vi "S2C_CMD_ShowCommand.vi"(7 "Error In":errorcluster, 10 "Row":i32, 11 "Data In":string[][](array[string])) -> (3 "Data Out":string[][](array[string]), 5 "Error Out":errorcluster)   [LabVIEW 2015]
doc: "Allows for the selection of available commands and parameters contained within a driver specific file."
panel:
  in  "Return":u16(ring) caption="Return Values"
  out "DriverText":string
  in  "Done":bool
  in  "Cmd":u16(ring) caption="Test"
  out "Init":bool
  in  "Params":i32(listbox) caption="Command"
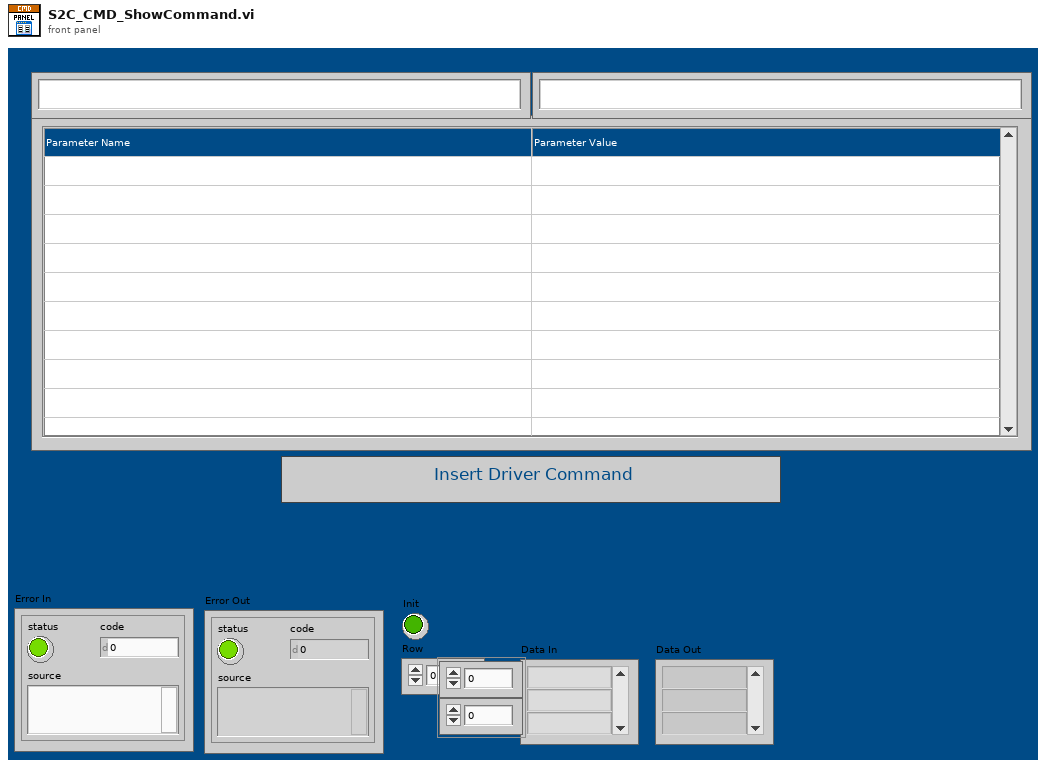
[diagram p1: front panel]
types:
  T1 = cluster{"Function":string, "Command":string, "Return":string, "Settings":string}
  T2 = typedef "LVPoint32TypeDef.ctl" = cluster{"Horizontal":i32, "Vertical":i32}
  T3 = typedef "LVRowAndColumnTypeDef.ctl" = cluster{"Row":i32, "Column":i32}
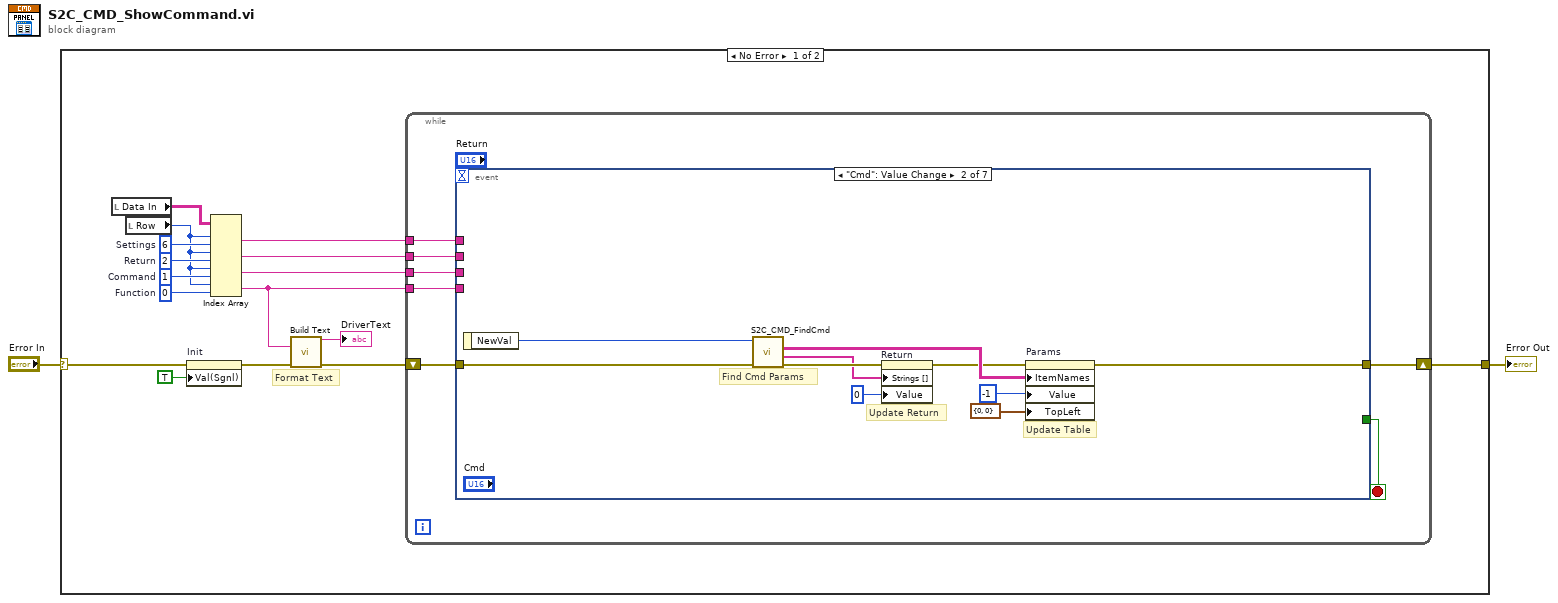
[diagram p0: block diagram]
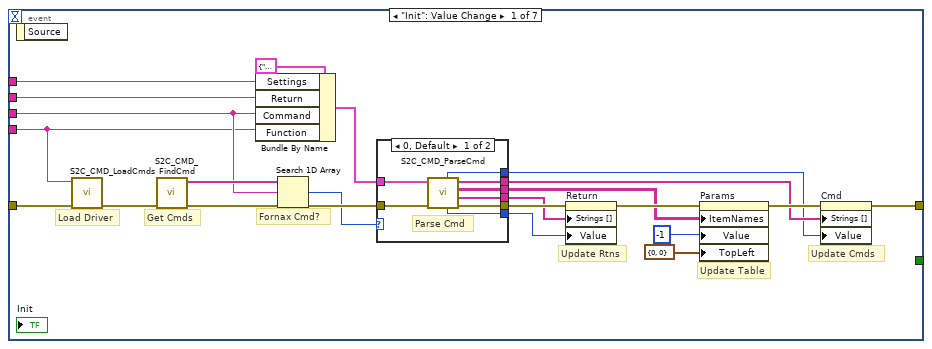
[diagram p2: hidden frame]
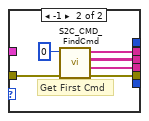
[diagram p3: hidden frame]
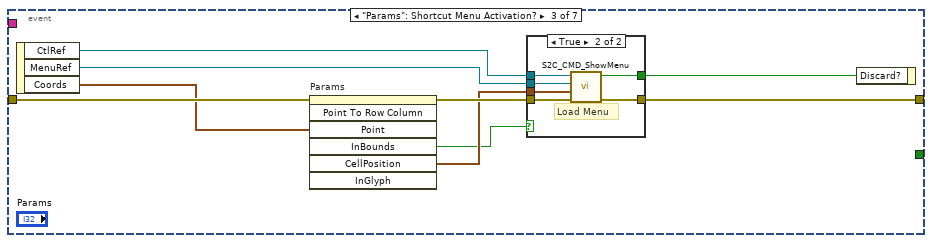
[diagram p4: hidden frame]
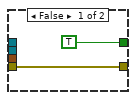
[diagram p5: hidden frame]
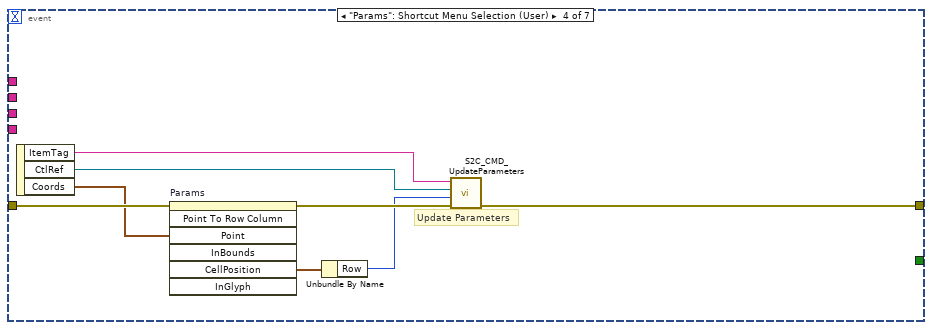
[diagram p6: hidden frame]
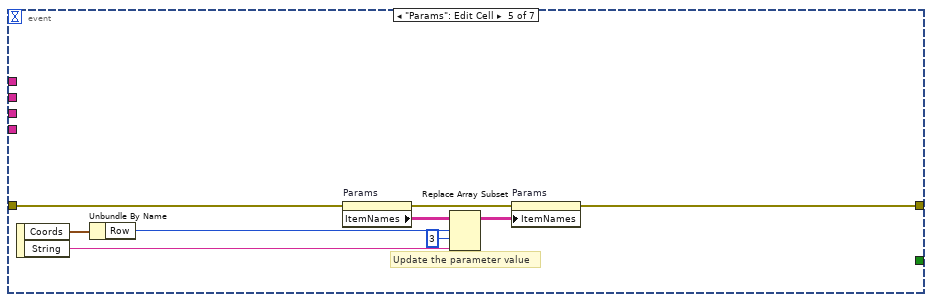
[diagram p7: hidden frame]
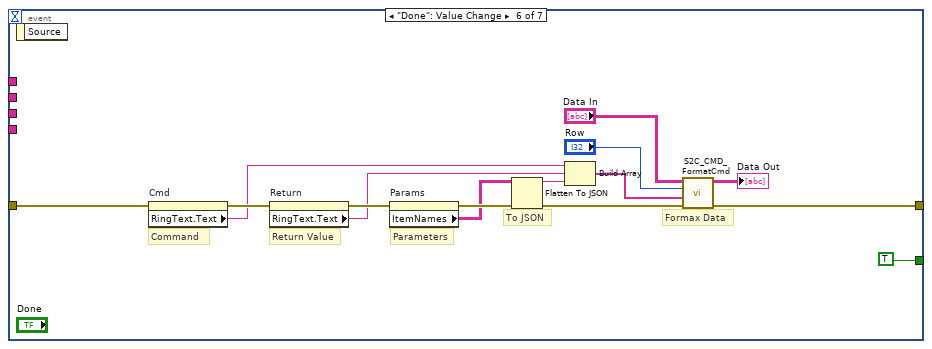
[diagram p8: hidden frame]
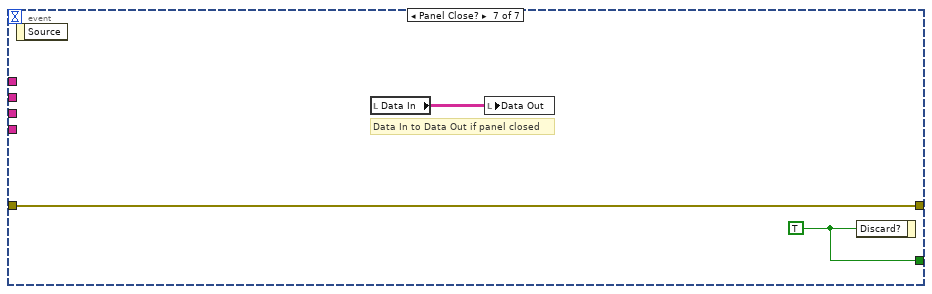
[diagram p9: hidden frame]
diagram:
  n1 = case shown="No Error" "Error In" {
    selector: "Error In" -> [w13 w124]
    tunnel: [w17 w124] -> w1
    frame No Error {
      w5 = 0  # Function
      w7 = 1  # Command
      w9 = 2  # Return
      w10 = 6  # Settings
      # "Format Text"
      n2 = local read "Data In"() -> (w15:string[][])
      n3 = local read "Row"() -> (w6:i32)
      n4 = property on="Init" class="Bool (strict)"(error in=w13, "Val(Sgnl)"=TRUE ("Value (Signaling)")) -> (error out=w12:errorcluster)  [unwired: 1 in, 1 out]
      n5 = Index Array(array=w15, index (row) #1=w6, index (col) #1=w10, index (row) #2=w6, index (col) #2=w9, index (row) #3=w6, index (col) #3=w7, index (row) #4=w6, index (col) #4=w5) -> (element #1=w14:string, element #2=w8:string, element #3=w3:string, element #4=w4:string)
      n6 = call "Build Text"("Driver"=w4, "error in (no error)"=w12) -> ("Result"=→"DriverText":string, "error out"=w11:errorcluster)  [unwired: 12 in]
      n7 = while {
        shift-right: [w24] -> w17
        shift-left: w11 -> [w25]
        tunnel: w14 -> [w22]
        tunnel: w8 -> [w21]
        tunnel: w4 -> [w20]
        tunnel: w3 -> [w19]
        stop <- w23 stop-if-true
        n8 = event shown="[1] \"Cmd\": Value Change" {
          selector: _ -> [_ _ _ _ _ _ _]
          dyn-events: _ -> [_ _ _ _ _ _ _]
          timeout: _ -> [_ _ _ _ _ _ _]
          tunnel: w25 -> [w41 w69 w80 w95 w104 w119 w123]
          tunnel: [w35 w70 w74 w93 w105 w108 w123] -> w24
          tunnel: [_ _ _ _ _ TRUE w122] -> w23
          tunnel: w22 -> [w31 _ _ _ _ _ _]
          tunnel: w21 -> [w30 _ _ _ _ _ _]
          tunnel: w20 -> [w28 _ _ _ _ _ _]
          tunnel: w19 -> [w29 _ _ _ _ _ _]
          event "Init": Value Change {
            # "Update Cmds"
            # "Load Driver"
            # "Fornax Cmd?"
            # "Get Cmds"
            # "Update Table"
            # "Update Rtns"
            n9 = event-data() -> ()  [unwired: 1 in, 1 out]
            n10 = call "S2C_CMD_LoadCmds.vi"("Error In"=w41, "Driver"=w28) -> ("Error Out"=w40:errorcluster)  [unwired: 9 in]
            n11 = call "S2C_CMD_FindCmd.vi"("Error In"=w40) -> ("Error Out"=w43:errorcluster, "AllCmds"=w34:string[])  [unwired: 7 in, 2 out]
            n12 = Bundle By Name(cluster=T1 {"Function"="", "Command"="", "Return"="", "Settings"=""}, "Settings"=w31, "Return"=w30, "Command"=w29, "Function"=w28) -> (w27:T1)
            n13 = Search 1D Array(1D array=w34, element=w29) -> (index of element=w42:i32)  [unwired: 1 in]
            n14 = case shown="0, Default" w42 {
              tunnel: w43 -> [w55 w61]
              tunnel: [w48 w56] -> w36
              tunnel: [w54 w59] -> w44
              tunnel: [w49 w57] -> w37
              tunnel: w27 -> [w53 _]
              tunnel: [w50 w58] -> w39
              tunnel: [w52 _] -> w32
              tunnel: [w51 _] -> w33
              frame 0, Default {
                # "Parse Cmd"
                n15 = call "S2C_CMD_ParseCmd.vi"("Error In"=w55, "Settings"=w53) -> ("Error Out"=w54:errorcluster, "Returns"=w50:string[], "Parameters"=w49:string[][], "Commands"=w48:string[], "RtnIndex"=w51:i32, "CmdIndex"=w52:i32)  [unwired: 4 in]
              }
              frame -1 {
                # "Get First Cmd"
                n16 = call "S2C_CMD_FindCmd.vi"("Error In"=w61, "Index"=0) -> ("Error Out"=w59:errorcluster, "Returns"=w58:string[], "Parameters"=w57:string[][], "AllCmds"=w56:string[])  [unwired: 6 in]
              }
            }
            n17 = property on="Return" class="Ring (strict)"(error in=w44, "Strings []"=w39, "Value"=w33) -> (error out=w45:errorcluster)  [unwired: 1 in, 1 out]
            n18 = property on="Params" class="MCListbox (strict)"(error in=w45, "ItemNames"=w37, "Value"=-1 ("Params"), "TopLeft"=cluster{"Row":u32, "Column":u32} {"Row"=0, "Column"=0} ("Top Left Visible Cell")) -> (error out=w38:errorcluster)  [unwired: 1 in, 1 out]
            n19 = property on="Cmd" class="Ring (strict)"(error in=w38, "Strings []"=w36, "Value"=w32) -> (error out=w35:errorcluster)  [unwired: 1 in, 1 out]
          }
          event "Cmd": Value Change {
            # "Update Return"
            # "Update Table"
            # "Find Cmd Params"
            n20 = event-data() -> ("NewVal"=w68:u16)  [unwired: 1 in]
            n21 = call "S2C_CMD_FindCmd.vi"("Error In"=w69, "Index"=w68) -> ("Error Out"=w65:errorcluster, "Returns"=w64:string[], "Parameters"=w67:string[][])  [unwired: 6 in, 1 out]
            n22 = property on="Return" class="Ring (strict)"(error in=w65, "Strings []"=w64, "Value"=u16 0) -> (error out=w63:errorcluster)  [unwired: 1 in, 1 out]
            n23 = property on="Params" class="MCListbox (strict)"(error in=w63, "ItemNames"=w67, "Value"=-1 ("Params"), "TopLeft"=cluster{"Row":u32, "Column":u32} {"Row"=0, "Column"=0} ("Top Left Visible Cell")) -> (error out=w70:errorcluster)  [unwired: 1 in, 1 out]
          }
          event "Params": Shortcut Menu Activation? {
            n24 = event-data() -> ("CtlRef"=w75:refnum<vi>, "MenuRef"=w76:refnum<k9>, "Coords"=w79:T2)  [unwired: 1 in]
            n25 = invoke on="Params" class="MCListbox (strict)" method="Point To Row Column"(error in=w80, "Point"=w79) -> (error out=w78:errorcluster, "InBounds"=w72:bool, "CellPosition"=w77:T3)  [unwired: 5 in, 4 out]
            n26 = case shown="True" w72 {
              tunnel: w78 -> [w82 w88]
              tunnel: w77 -> [_ w87]
              tunnel: w76 -> [_ w86]
              tunnel: w75 -> [_ w85]
              tunnel: [w82 w84] -> w74
              tunnel: [TRUE ("Discard?") w83] -> w73
              frame False {
              }
              frame True {
                # "Load Menu"
                n27 = call "S2C_CMD_ShowMenu.vi"("Error In"=w88, "Cell Position"=w87, "MenuRef"=w86, "CtlRef"=w85) -> ("Error Out"=w84:errorcluster, "Discard?"=w83:bool)  [unwired: 6 in]
              }
            }
            n28 = event-data("Discard?"=w73) -> ()  [unwired: 1 in, 1 out]
          }
          event "Params": Shortcut Menu Selection (User) {
            # "Update Parameters"
            n29 = event-data() -> ("ItemTag"=w90:string, "CtlRef"=w89:refnum<vi>, "Coords"=w91:T2)  [unwired: 1 in]
            n30 = invoke on="Params" class="MCListbox (strict)" method="Point To Row Column"(error in=w95, "Point"=w91) -> (error out=w94:errorcluster, "CellPosition"=w96:T3)  [unwired: 5 in, 5 out]
            n31 = Unbundle By Name(w96) -> ("Row"=w92:i32)
            n32 = call "S2C_CMD_UpdateParameters.vi"("Error In"=w94, "Row"=w92, "CtlRef"=w89, "ItemTag"=w90) -> ("Error Out"=w93:errorcluster)  [unwired: 7 in]
          }
          event "Params": Edit Cell {
            # "Update the parameter value"
            n33 = event-data() -> ("Coords"=w103:T3, "String"=w98:string)  [unwired: 1 in]
            n34 = Unbundle By Name(w103) -> ("Row"=w99:i32)
            n35 = property on="Params" class="MCListbox (strict)"(error in=w104) -> (error out=w97:errorcluster, "ItemNames"=w101:string[][])  [unwired: 1 in, 1 out]
            n36 = Replace Array Subset(array=w101, new element=w98, index (row)=w99, index (col)=3 ("disabled index (col)")) -> (w100:string[][])
            n37 = property on="Params" class="MCListbox (strict)"(error in=w97, "ItemNames"=w100) -> (error out=w105:errorcluster)  [unwired: 1 in, 1 out]
          }
          event "Done": Value Change {
            # "Formax Data"
            # "To JSON"
            # "Parameters"
            # "Return Value"
            # "Command"
            n38 = event-data() -> ()  [unwired: 1 in, 1 out]
            n39 = property on="Cmd" class="Ring (strict)"(error in=w119) -> (error out=w118:errorcluster, "RingText.Text"=w114:string)  [unwired: 1 in, 1 out]
            n40 = property on="Return" class="Ring (strict)"(error in=w118) -> (error out=w117:errorcluster, "RingText.Text"=w113:string)  [unwired: 1 in, 1 out]
            n41 = property on="Params" class="MCListbox (strict)"(error in=w117) -> (error out=w116:errorcluster, "ItemNames"=w115:string[][])  [unwired: 1 in, 1 out]
            n42 = Flatten To JSON(anything=w115, error in (no error)=w116) -> (JSON string=w106:string, 11:w112:errorcluster)  [unwired: 1 in]
            n43 = Build Array(w114, w113, w106) -> (w111:string[])
            n44 = call "S2C_CMD_FormatCmd.vi"("Error In"=w112, "TableData"=w111, "Row"="Row", "Data In"="Data In") -> ("Error Out"=w108:errorcluster, "Data Out"=→"Data Out":string[][])  [unwired: 6 in]
          }
          event Panel Close? {
            w122 = TRUE
            # "Data In to Data Out if panel closed"
            n45 = event-data() -> ()  [unwired: 1 in, 1 out]
            n46 = local read "Data In"() -> (w121:string[][])
            n47 = local write "Data Out"(w121) -> ()
            n48 = event-data("Discard?"=w122) -> ()  [unwired: 1 in, 1 out]
          }
        }
      }
    }
    frame Error {
    }
  }
  "Error Out" <- w1
